vi "Insert Error.vi"(0 "[error code] (0)":i32 format="%0.0f", 2 "error description":string, 3 "error in (no error)":errorcluster, 4 "error?":bool) -> (10 "error out":errorcluster)   [LabVIEW 2014, in "Utilities.lvlib"]
uses:
  Utilities.lvlib
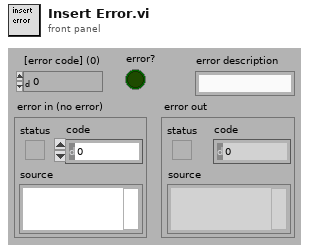
[diagram p1: front panel]
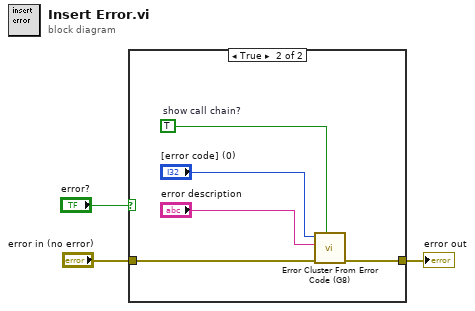
[diagram p0: block diagram]
diagram:
  n1 = case shown="True" "error?" {
    tunnel: "error in (no error)" -> [w4 w9]
    tunnel: [w4 w8] -> w2
    frame False {
    }
    frame True {
      w5 = TRUE  # show call chain?
      n2 = call "Error Cluster From Error Code (G8).vi"("show call chain? (False)"=w5, "error in (no error)"=w9, "error message (\"\")"="error description", "error code (0)"="[error code] (0)") -> ("error out"=w8:errorcluster)  [unwired: 5 in]
    }
  }
  "error out" <- w2
